vi "Subvi pixel clock.vi"(10 "Memory label":refnum<k21>="Pixel clock buffer") -> ()   [LabVIEW 2017]
uses:
  <vilib>/rvi/Emulation/niFpgaSctlEmulationGetInTimedLoop.vi
  <vilib>/rvi/DataTransferAndStorage/Container/Common/niFpgaContainerExecOnDevCompGetState.vi
  <vilib>/rvi/Emulation/niFpgaEmulationIsFPGAContextNoSignature.vi
  <vilib>/rvi/DataTransferAndStorage/Container/Common/niFpgaContainerGetUniqueNameForEmu.vi
  <vilib>/rvi/Emulation/niFpgaProcessEmulError.vi
  <vilib>/rvi/errors/nirviReportUnexpectedCaseInternalError (U32).vi
  <vilib>/rvi/Memory/Memory_Emulation/niFpgaMemoryEmulationCacheClearOnFirstRun.vi
  <vilib>/rvi/Memory/Memory_Emulation/nirvimemoryEmulationManagerCache_MakeExclusive.vi
  <vilib>/rvi/Memory/Memory_Emulation/niFpgaMemoryEmulationValidateCache.vi
  <vilib>/rvi/Memory/Memory_Emulation/nirvimemoryEmulationManagerCache_InsertValue.vi
  <vilib>/Utility/error.llb/Clear Errors.vi
  <vilib>/rvi/Memory/Memory_Emulation/nirvimemoryEmulationManagerCache_ReleaseExclusive.vi
  <vilib>/rvi/Memory/Memory_Emulation/nirvimemoryEmulationManagerCache_GetValue.vi
  <vilib>/rvi/Memory/Memory_Emulation/nirvimemoryEmulationManagerCache_SetValue.vi
  <vilib>/rvi/Emulation/niFpgaSctlEmulationResourceMgr.vi
  Detector/GV pixel clock.vi
  Detector/GV N pixel clock per line.vi
  <vilib>/rvi/DataTransferAndStorage/Container/XNode/niFpgaContainer.xnode
  <vilib>/rvi/Memory/Memory_Emulation/niFpgaMemoryEmulationRefIn.vi
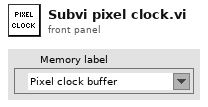
[diagram p1: front panel]
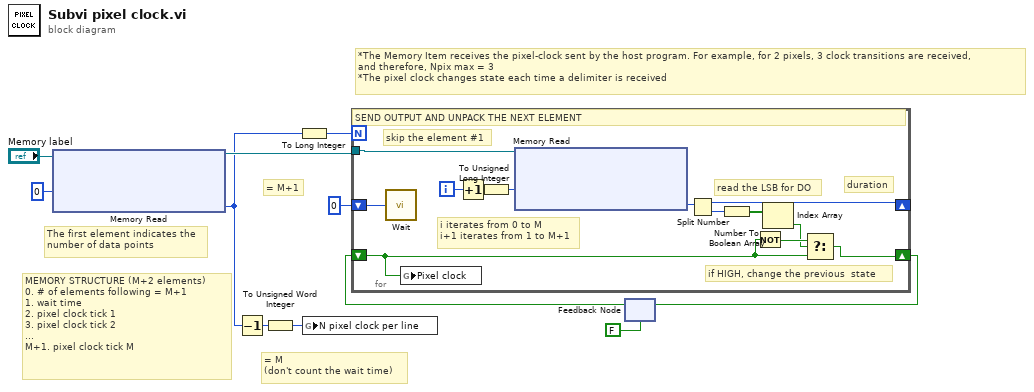
[diagram p0: block diagram]
diagram:
  # "= M+1"
  # "= M\n(don't count the wait time)"
  # "MEMORY STRUCTURE (M+2 elements)\n0. # of elements following = M+1\n1. wait time\n2. pixel clock tick 1\n3. pixel clock tick 2\n...\nM+1. pixel clock tick M"
  # "*The Memory Item receives the pixel-clock sent by the host program. For example, for 2 pixels, 3 clock transitions are received, \nand therefore, Npix max = 3\n*The pixel clock changes state each time a delimiter is received"
  # "The first element indicates the\nnumber of data points"
  n1 = xnode ("Memory Read")("Address"=u32 0, "Memory In"="Memory label") -> ("Data"=w5:u32, "Memory Out"=w11:refnum<k21>)
  n2 = Decrement(x=w5) -> (x-1=w4:u32)
  n3 = To Unsigned Word Integer(number=w4) -> (unsigned 16bit integer=w3:u16)
  n4 = To Long Integer(number=w5) -> (32bit integer=w2:i32)
  n5 = global write "GV N pixel clock per line.vi" "N pixel clock per line"(w3) -> ()
  n6 = feedback #1(FALSE) -> (w7:bool)
  n7 = for {
    N: w2 -> [_]
    shift-right: [w17] -> w8
    shift-left: w7 -> [w12]
    tunnel: w11 -> [w21]
    shift-right: [w15] -> _
    shift-left: u16 0 -> [w16]
    i -> [w23]
    # "i iterates from 0 to M\ni+1 iterates from 1 to M+1"
    # "skip the element #1"
    # "if HIGH, change the previous  state"
    # "read the LSB for DO"
    # "duration"
    # "SEND OUTPUT AND UNPACK THE NEXT ELEMENT"
    n8 = call "Wait"("Count(Ticks)"=w16) -> ()  [unwired: 1 out]
    n9 = global write "GV pixel clock.vi" "Pixel clock"(w12) -> ()
    n10 = Increment(x=w23) -> (x+1=w22:i32)
    n11 = To Unsigned Long Integer(number=w22) -> (unsigned 32bit integer=w13:u32)
    n12 = xnode ("Memory Read")("Address"=w13, "Memory In"=w21) -> ("Data"=w24:u32)  [unwired: 1 out]
    n13 = Split Number(x=w24) -> (hi(x)=w15:u16, lo(x)=w19:u16)
    n14 = Number To Boolean Array(number=w19) -> (Boolean array=w20:bool[])
    n15 = Not(x=w12) -> (.not. x?=w18:bool)
    n16 = Index Array(array=w20) -> (element=w14:bool)  [unwired: 1 in]
    n17 = Select(t=w18, s=w14, f=w12) -> (s? t:f=w17:bool)
  }
  n18 = feedback-in #1(w8) -> ()
